vi "DeviceOff.vi"(8 "error in (no error)":errorcluster, 11 "NHRDCModel in":refnum<class "NHRDCPowerModel.lvclass">) -> (0 "error out":errorcluster, 3 "NHRDCModel out":refnum<class "NHRDCPowerModel.lvclass">)   [LabVIEW 2018, in "AcPwrPlugins.lvlib" / "NHRDCPowerModel.lvclass"]
doc: "This VI disables the instruments output form either generating or receiving a signal."
uses:
  NHRDCPowerModel.lvclass
  NHRDCPowerClass/NHRDCPower.lvclass
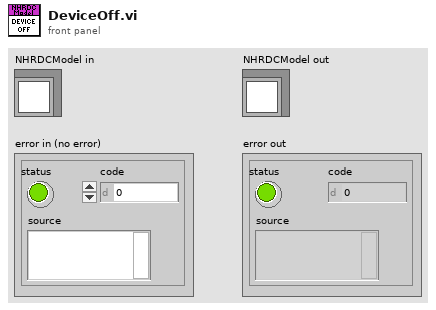
[diagram p1: front panel]
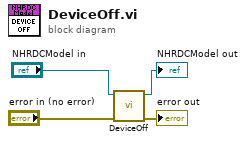
[diagram p0: block diagram]
diagram:
  n1 = call-parent "DeviceOff.vi"("error in (no error)"="error in (no error)", "NHRDCPower in"="NHRDCModel in") -> ("error out"=→"error out":errorcluster, "NHRDCPower out"=→"NHRDCModel out":refnum<class "NHRDCPowerModel.lvclass">)  [unwired: 8 in]
